vi "Analyse.vi"() -> ()   [LabVIEW 2017]
uses:
  C:/Users/h16034903/Downloads/Masure_Henry_projet.llb/Variable globale 1.vi
panel:
  in  "cluster de sortie 2":T1
  out "Commentaire : veuillez déplacer le curseur bleu":string
  out "Amplitude du signal":dbl
  out "Intervalle de temps":dbl
  in  "stop":bool
  out "Informations d'enregistrement":T2
  out "Informations du patient":T3
  out "Graphe":dbl[][](graph)
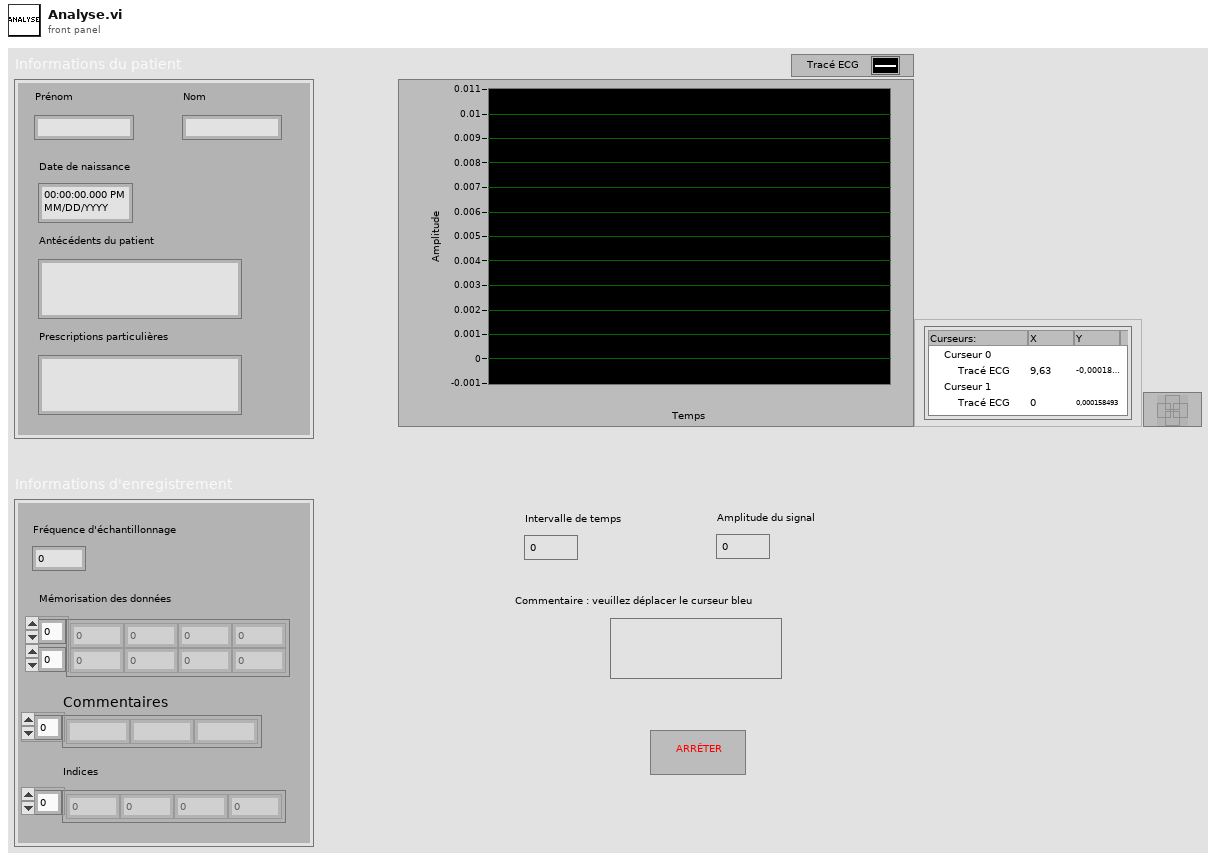
[diagram p1: front panel]
types:
  T1 = cluster{"frequence echantillonage":dbl, "ECG filtré\n":dbl[][], string[], "Nom":string, "Prénom":string, "Date de l'examen":timestamp, i32[]}
  T2 = cluster{"Fréquence d'échantillonnage":dbl, "Mémorisation des données\n":dbl[][], "Commentaires":string[], "Indices":dbl[]}
  T3 = cluster{"Prénom":string, "Nom":string, "Date de naissance":timestamp, "Antécédents du patient":string, "Prescriptions particulières":string}
  T4 = cluster{"frequence echantillonage":dbl, "ECG filtré\n":dbl[][], string[], i32[]}
  T5 = cluster{"Nom":string, "Prénom":string, "Date de l'examen":timestamp, "Antécédents du patient":string, "Prescriptions particulières":string}
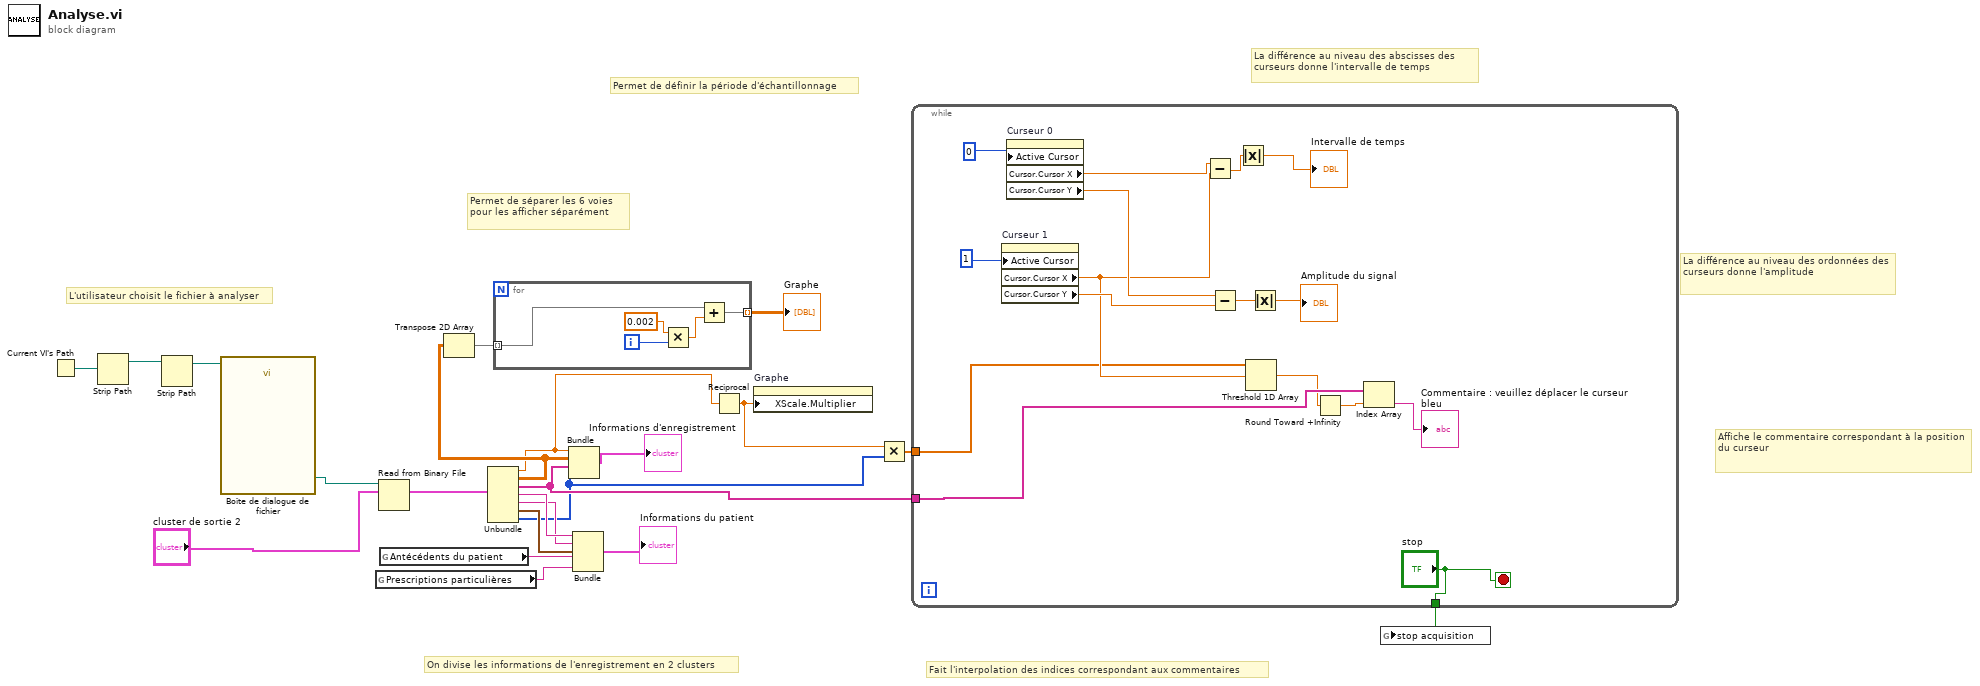
[diagram p0: block diagram]
diagram:
  # "Affiche le commentaire correspondant à la position du curseur"
  # "La différence au niveau des ordonnées des curseurs donne l'amplitude"
  # "La différence au niveau des abscisses des curseurs donne l'intervalle de temps"
  # "Permet de définir la période d'échantillonnage"
  # "On divise les informations de l'enregistrement en 2 clusters"
  # "Fait l'interpolation des indices correspondant aux commentaires"
  # "Permet de séparer les 6 voies pour les afficher séparément"
  # "L'utilisateur choisit le fichier à analyser"
  n1 = Current VI's Path() -> (path=w19:path)
  n2 = Strip Path(path=w19) -> (stripped path=w18:path)  [unwired: 1 out]
  n3 = Strip Path(path=w18) -> (stripped path=w17:path)  [unwired: 1 out]
  n4 = call "Boîte de dialogue de fichier"("start path"=w17) -> ("selected path"=w20:path)  [unwired: 11 in, 3 out]
  n5 = global read "Variable globale 1.vi" "Prescriptions particulières"() -> (w8:string)
  n6 = Read from Binary File(5:"cluster de sortie 2", 11:w20) -> (2:w15:T1)  [unwired: 4 in, 3 out]
  n7 = global read "Variable globale 1.vi" "Antécédents du patient"() -> (w9:string)
  n8 = Unbundle(w15) -> ("frequence echantillonage"=w5:dbl, "ECG filtré"=w12:dbl[][], w7:string[], "Nom"=w22:string, "Prénom"=w21:string, "Date de l'examen"=w10:timestamp, w3:i32[])
  n9 = Transpose 2D Array(2D array=w12) -> (transposed array=w16:dbl[][])
  n10 = for {
    tunnel: w16 -> [w23] mode=indexing
    tunnel: [w24] -> w14 mode=indexing
    i -> [w25]
    n11 = Multiply(x=0.002, y=w25) -> (x*y=w26:dbl)
    n12 = Add(x=w23, y=w26) -> (x+y=w24:dbl[])
  }
  "Graphe" <- w14
  n13 = Bundle("frequence echantillonage"=w5, "ECG filtré"=w12, w7, w3) -> (→"Informations d'enregistrement":T4)  [unwired: 1 in]
  n14 = Bundle("Nom"=w22, "Prénom"=w21, "Date de l'examen"=w10, "Antécédents du patient"=w9, "Prescriptions particulières"=w8) -> (→"Informations du patient":T5)  [unwired: 1 in]
  n15 = Reciprocal(x=w5) -> (1/x=w2:dbl)
  n16 = property on="Graphe" class="GraphWF (strict)"("XScale.Multiplier"=w2) -> ()  [unwired: 2 in, 2 out]
  n17 = Multiply(x=w2, y=w3) -> (x*y=w4:dbl[])
  n18 = while {
    tunnel: w7 -> [w34]
    tunnel: w4 -> [w31]
    tunnel: ["stop"] -> w1
    stop <- "stop" stop-if-true
    n19 = property on="Curseur 1" class="GraphWF (strict)"("Active Cursor"=u32 1 ("Curseur actif")) -> ("Cursor.Cursor X"=w32:dbl, "Cursor.Cursor Y"=w37:dbl)  [unwired: 2 in, 2 out]
    n20 = property on="Curseur 0" class="GraphWF (strict)"("Active Cursor"=u32 0 ("Curseur actif")) -> ("Cursor.Cursor X"=w41:dbl, "Cursor.Cursor Y"=w38:dbl)  [unwired: 2 in, 2 out]
    n21 = Subtract(x=w41, y=w32) -> (x-y=w40:dbl)
    n22 = Subtract(x=w38, y=w37) -> (x-y=w36:dbl)
    n23 = Absolute Value(x=w40) -> (abs(x)=→"Intervalle de temps":dbl)
    n24 = Threshold 1D Array(2:w32, 3:w31) -> (0:w30:dbl)  [unwired: 1 in]
    n25 = Absolute Value(x=w36) -> (abs(x)=→"Amplitude du signal":dbl)
    n26 = Round Toward +Infinity(x=w30) -> (ceil(x): smallest int >= x=w29:dbl)
    n27 = Index Array(array=w34, index=w29) -> (element=→"Commentaire : veuillez déplacer le curseur bleu":string)
  }
  n28 = global write "Variable globale 1.vi" "stop acquisition"(w1) -> ()
